vi "Enable Add Delete.vi"(5 "Delete Ref":refnum<vi>, 7 "Add Ref":refnum<vi>, 8 "error in (no error)":errorcluster, 11 "Slider Ref Array":refnum<vi>[](array[refnum])) -> (0 "error out":errorcluster)   [LabVIEW 2017, in "3D Plot.lvclass"]
uses:
  <vilib>/Math Plots/3D Math Plots/3D Plot/3D Plot/3D Plot.lvclass
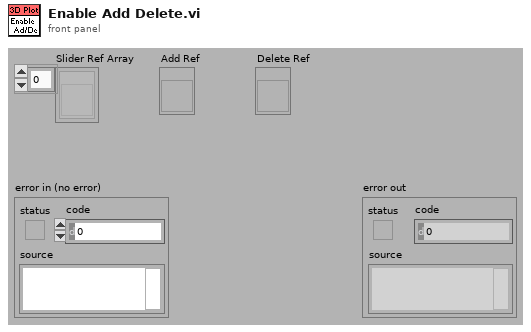
[diagram p1: front panel]
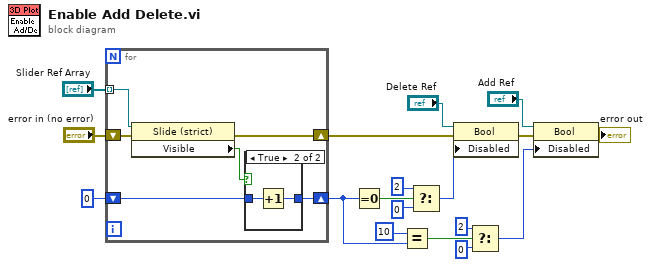
[diagram p0: block diagram]
diagram:
  n1 = for {
    tunnel: "Slider Ref Array" -> [w24] mode=indexing
    shift-right: [w21] -> w13
    shift-left: 0 -> [w22]
    shift-right: [w19] -> w3
    shift-left: "error in (no error)" -> [w20]
    n2 = property on="Property Node" class="Slide (strict)"(reference=w24, error in=w20) -> (error out=w19:errorcluster, "Visible"=w23:bool)  [unwired: 1 out]
    n3 = case shown="True" w23 {
      tunnel: w22 -> [w25 w27]
      tunnel: [w25 w26] -> w21
      frame False {
      }
      frame True {
        n4 = Increment(x=w27) -> (x+1=w26:i32)
      }
    }
  }
  n5 = Equal To 0?(x=w13) -> (x = 0?=w12:bool)
  n6 = Equal?(x=10, y=w13) -> (x = y?=w6:bool)
  n7 = Select(t=u8 2, s=w12, f=u8 0 ("t")) -> (s? t:f=w9:u8)
  n8 = property on="Property Node" class="Bool"(reference="Delete Ref", error in=w3, "Disabled"=w9) -> (error out=w2:errorcluster)  [unwired: 1 out]
  n9 = Select(t=u8 2, s=w6, f=u8 0 ("t")) -> (s? t:f=w5:u8)
  n10 = property on="Property Node" class="Bool"(reference="Add Ref", error in=w2, "Disabled"=w5) -> (error out=→"error out":errorcluster)  [unwired: 1 out]
